vi "Investigate SCTL Errors.vi"() -> ()   [LabVIEW 2010]
uses:
  <vilib>/eio/EIONode/EIONode.xnode
  <vilib>/Platform/TimedLoop/XDataNode/XDataNode.xnode
  <vilib>/Platform/TimedLoop/XDataNode/nitl_modes.ctl
  <vilib>/Platform/TimedLoop/XDataNode/XDNodeRunTimeDep.lvlib
  <vilib>/Platform/TimedLoop/XDataNode/wakeup.ctl
  <vilib>/Platform/TimedLoop/XDataNode/timing_clust.ctl
panel:
  in  "stop":bool
  out "Average Acceleration":fxp<+/-,53,27> format="%.35g"
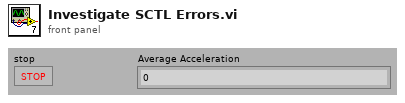
[diagram p1: front panel]
types:
  T1 = typedef "XDNodeRunTimeDep.lvlib/timing_clust.ctl" = cluster{"Expected End [f-1]":u64, "Actual End [f-1]":u64, "Finished Late? [f-1]":bool, "Expected End [i-1]":u64, "Actual End [i-1]":u64, "Finished Late? [i-1]":bool, "Expected Start [i]":u64, "Actual Start [i]":u64, "Expected Start [f]":u64, "Actual Start [f]":u64, "Source Name":string, "Structure Name":string, "Period":i64, "Deadline":i64, "Offset":i64, "Start":i64, "Priority":i32, "Timeout":i32, "Mode":T2, "Wakeup Reason":T3, "Error":errorcluster, "Source Type":string, "Secondary Source Type":string, "Global End Time":u64, "Global Start Time":u64, "Frame Duration":u64, "Iteration Duration":u64, "Assigned CPU":i32, "I/O Scan Engine Mode":u32}
  T2 = typedef "XDNodeRunTimeDep.lvlib/nitl_modes.ctl" = enum32{"No Change", "Process missed periods, maintain original phase", "Discard missed periods, maintain original phase", "Process missed periods, ignore original phase", "Discard missed periods, ignore original phase"}
  T3 = typedef "XDNodeRunTimeDep.lvlib/wakeup.ctl" = enum32{"Normal", "Aborted", "Asynchronous wakeup", "Timing source error", "Timed loop error", "Timeout"}
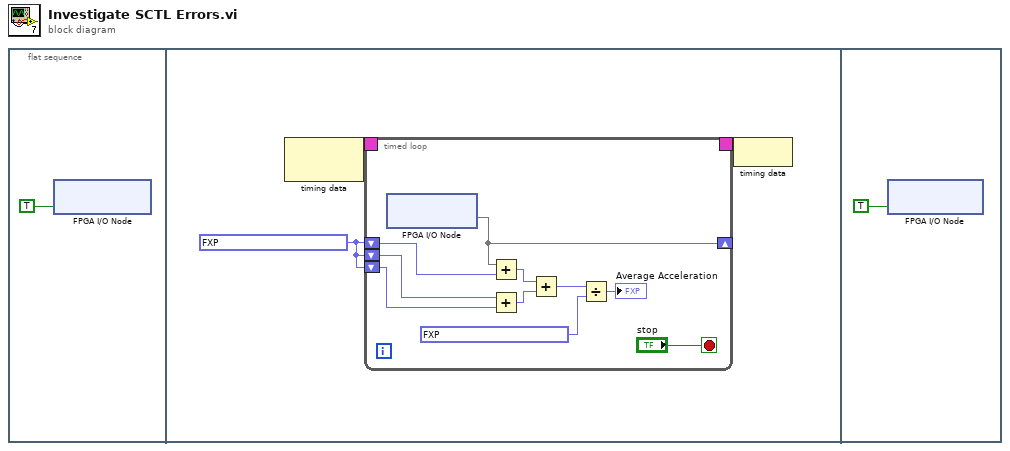
[diagram p0: block diagram]
diagram:
  n1 = flat-sequence {
    frame #0 {
      n2 = xnode "FPGA I/O Node"("Mod2/Start"=TRUE) -> ()  [unwired: 1 in, 1 out]
    }
    frame #1 {
      w2 = fxp<+/-,24,4> 0.0 ("Mod2/AI0")
      n3 = node-c288() -> (w4:T1)  [unwired: 1 in]
      n4 = timed-loop {
        timing: w4 -> [_]
        timing-out: [_] -> w3
        shift-right: [w5] -> _
        shift-left: w2 -> [w12]
        shift-left: w2 -> [w11]
        shift-left: w2 -> [w10]
        stop <- "stop" stop-if-true
        n5 = xnode "FPGA I/O Node"() -> ("Mod2/AI0"=w5)  [unwired: 1 in, 1 out]
        n6 = Add(x=w5, y=w12) -> (x+y=w14:fxp<+/-,25,5>)
        n7 = Add(x=w11, y=w10) -> (x+y=w13:fxp<+/-,25,5>)
        n8 = Add(x=w14, y=w13) -> (x+y=w9:fxp<+/-,26,6>)
        n9 = Divide(x=w9, y=fxp<+/-,26,6> 4.0) -> (x/y=→"Average Acceleration":fxp<+/-,53,27>)
      }
      n10 = node-c288(w3) -> ()
    }
    frame #2 {
      n11 = xnode "FPGA I/O Node"("Mod2/Stop"=TRUE) -> ()  [unwired: 1 in, 1 out]
    }
  }
